vi "Allocate FFT Library.vi"(8 "Error In":errorcluster) -> (0 "Error Out":errorcluster)   [LabVIEW 2012, in "OpenCLV x64.lvlib"]
doc: "Inits and Allocates the FFT Library"
uses:
  OpenCLV x64.lvlib
  Error Checking/Add Error Functional Global.vi
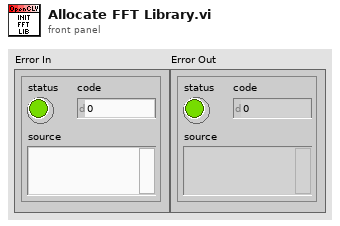
[diagram p1: front panel]
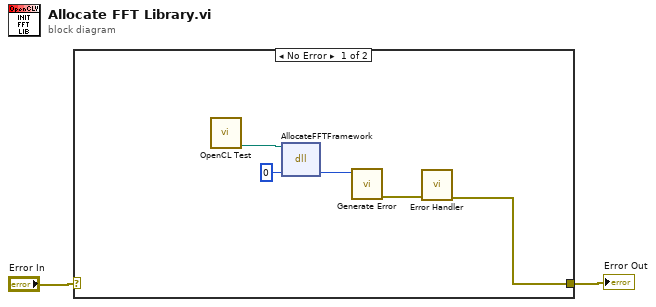
[diagram p0: block diagram]
diagram:
  n1 = case shown="No Error" "Error In" {
    selector: "Error In" -> [_ w8]
    tunnel: [w3 w8] -> w1
    frame No Error {
      n2 = call "OpenCL Test.vi"() -> ("DLL To Use"=w5:path)  [unwired: 11 in]
      n3 = dll-call lib="?" fn="AllocateFFTFramework"(path in=w5, "Error"=0) -> ("Error"=w6:i32)  [unwired: 3 in, 2 out]
      n4 = call "Generate Error.vi"("Error"=w6) -> ("error out"=w4:errorcluster)  [unwired: 10 in]
      n5 = call-poly "Error Handler.vi"("Error In"=w4) -> ("Error Out"=w3:errorcluster)  [unwired: 10 in]
    }
    frame Error {
    }
  }
  "Error Out" <- w1
